vi "ValueAtNearestTimestamp.vi"(9 "Values":dbl[](array[numeric]), 10 "SelectedTimestamp":dbl format="%#_13g", 11 "TimeStamps":dbl[](array[numeric]) format="%#_12g") -> (1 "ValueAtClosestIndex":dbl, 2 "ClosestMatchIndex":i32)   [LabVIEW 2018]
doc: "Given the array of timestamps and corresponding array of values, scan through the timestamp array and find the closest one to Selected Timestamp. Output the index of that timestamp and the corresponding value from the Values array."
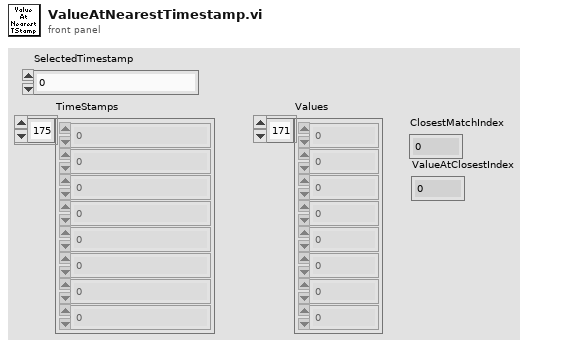
[diagram p1: front panel]
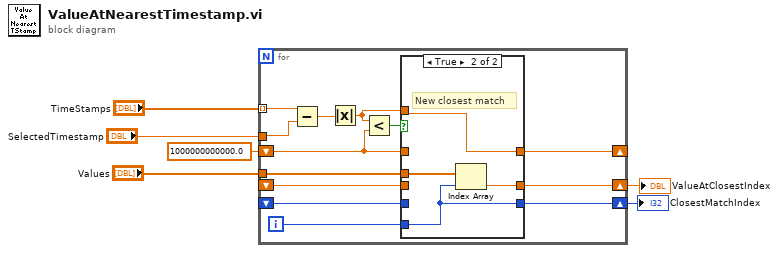
[diagram p0: block diagram]
diagram:
  n1 = for {
    tunnel: "TimeStamps" -> [w19] mode=indexing
    tunnel: "SelectedTimestamp" -> [w18]
    shift-right: [w15] -> _
    shift-left: 1000000000000.0 -> [w7]
    shift-right: [w12] -> w2
    shift-left: _ -> [w11]
    shift-right: [w9] -> w1
    shift-left: _ -> [w8]
    tunnel: "Values" -> [w10]
    i -> [w13]
    n2 = Subtract(x=w19, y=w18) -> (x-y=w17:dbl)
    n3 = Absolute Value(x=w17) -> (abs(x)=w14:dbl)
    n4 = Less?(x=w14, y=w7) -> (x < y?=w16:bool)
    n5 = case shown="True" w16 {
      tunnel: [w20 w26] -> w15
      tunnel: w14 -> [_ w26]
      tunnel: w13 -> [_ w24]
      tunnel: [w22 w24] -> w12
      tunnel: w11 -> [w22 _]
      tunnel: w10 -> [_ w25]
      tunnel: [w21 w23] -> w9
      tunnel: w8 -> [w21 _]
      tunnel: w7 -> [w20 _]
      frame False {
      }
      frame True {
        # "New closest match"
        n6 = Index Array(array=w25, index=w24) -> (element=w23:dbl)
      }
    }
  }
  "ClosestMatchIndex" <- w2
  "ValueAtClosestIndex" <- w1
